vi "LEDtest.vi"() -> ()   [LabVIEW 2012]
uses:
  <vilib>/userdefined/High Color/nirio_resource_hc.ctl
  <vilib>/FPGAPlugInAG/PXI-7951R/niLvFpga_Open_PXI-7951R.vi
  <vilib>/rvi/interface/common/dynamic/niFpgaDynamicAddResources.vi
  <vilib>/FPGAPlugInAG/Dynamic/niLvFpga_Reset_Dynamic.vi
  <vilib>/Utility/error.llb/Error Cluster From Error Code.vi
  <vilib>/rvi/errors/niLvFpgaAdjustHostInterfaceError.vi
  <vilib>/FPGAPlugInAG/Dynamic/niLvFpga_Run_Dynamic.vi
  <vilib>/FPGAPlugInAG/Dynamic/niLvFpga_Close_Dynamic.vi
  <vilib>/rvi/interface/nirviOpenFPGA/nirviOpenFPGA.xnode
  FPGA Bitfiles/ModuDAQ_FPGATarget_testrandled_sOjUljTr4qA.lvbitx
  <vilib>/rvi/interface/nirviMethod/nirviMethod.xnode
  <vilib>/rvi/interface/nirviReadWriteControl/nirviReadWriteControl.xnode
  <vilib>/rvi/interface/nirviCloseFPGA/nirviCloseFPGA.xnode
  <vilib>/rvi/interface/Simulation/niFpgaSimulationCallBeginRW.vi
  NiFpgaLv.dll
panel:
  out "error out":errorcluster
  out "Wait counter":u32
  out "Total number of pulses sent":u64
  out "Is Test Pulse?":bool
  in  "Testpulse Time Delay (20 ns ticks)":u32=14
  in  "Pulse duration (us)":u32=5
  in  "resource name":T1 caption="RIO Device"
  in  "stop":bool
  in  "LED On":bool
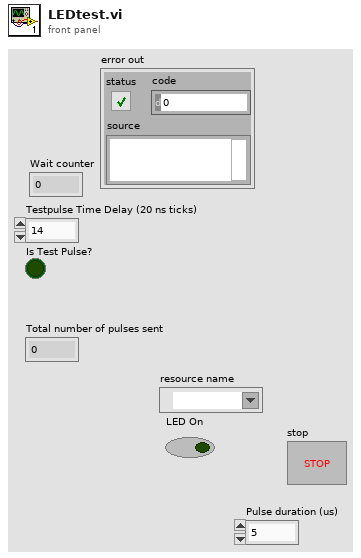
[diagram p1: front panel]
types:
  T1 = typedef "nirio_resource_hc.ctl" = tag
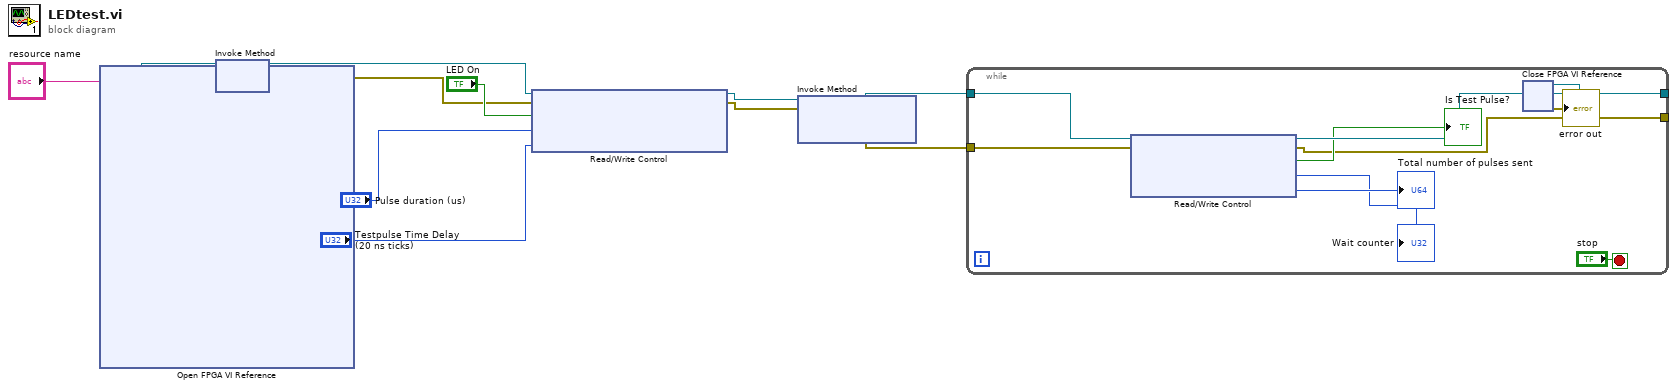
[diagram p0: block diagram]
diagram:
  n1 = xnode "Open FPGA VI Reference"("resource name"="resource name") -> ("FPGA VI Reference Out"=w4:refnum<k20>, "error out"=w3:errorcluster)  [unwired: 1 in]
  n2 = xnode "Invoke Method"("FPGA VI Reference In"=w4, "error in"=w3) -> ("FPGA VI Reference Out"=w2:refnum<k20>, "error out"=w1:errorcluster)
  n3 = xnode "Read/Write Control"("FPGA VI Reference In"=w2, "error in"=w1, "Testpulser On/Off"="LED On", "Testpulse duration (20 ns ticks)"="Pulse duration (us)", "Testpulse Time Delay (20 ns ticks)"="Testpulse Time Delay (20 ns ticks)") -> ("FPGA VI Reference Out"=w8:refnum<k20>, "error out"=w7:errorcluster)
  n4 = xnode "Invoke Method"("FPGA VI Reference In"=w8, "error in"=w7) -> ("FPGA VI Reference Out"=w6:refnum<k20>, "error out"=w5:errorcluster)  [unwired: 1 in]
  n5 = while {
    tunnel: [w22] -> w14
    tunnel: w6 -> [w21]
    tunnel: w5 -> [w17]
    tunnel: [w16] -> w10
    stop <- "stop" stop-if-true
    n6 = xnode "Read/Write Control"("FPGA VI Reference In"=w21, "error in"=w17) -> ("FPGA VI Reference Out"=w22:refnum<k20>, "error out"=w16:errorcluster, "Is Test Pulse?"=→"Is Test Pulse?":bool, "Wait counter"=→"Wait counter":u32, "Total number of pulses sent"=→"Total number of pulses sent":u64)
  }
  n7 = xnode "Close FPGA VI Reference"("FPGA VI Reference In"=w14, "error in"=w10) -> ("error out"=→"error out":errorcluster)
